vi "PPG_ABC.constructor.vi"(0 "name":string, 2 "data in":string, 5 "error in(no error)":errorcluster) -> (14 "i ref out":refnum<vi>, 16 "data out":string, 19 "error out":errorcluster)   [LabVIEW 2014, in "PPG_ABC.lvlib"]
doc: "This is the constructor of a class.\n\nLicense Agreement for this software:\n\nCopyright (C)\nGesellschaft für Schwerionenforschung, GSI\nPlanckstr. 1\n64291 Darmstadt\nGermany\n\nContact: D.Beck@gsi.de \n\nThis program is free software; you can redistribute it and/or modify it under the terms of the \nGNU General Public License as published by the Free Software Foundation; either version 2 of \nthe license, or (at your option) any later version.\n\nThis program is distributed in the hope that it will be useful, but WITHOUT ANY WARRANTY; \nwithout even the implied warranty of MERCHANTABILITY or FITNESS FOR A PARTICULAR PURPOSE. See the GNU General License for more details (http://www.gnu.org).\n\nGesellschaft für Schwerionenforschung, GSI\nPlanckstr. 1, 64291 Darmstadt, Germany\nFor all questions and ideas contact: M.Richter@gsi.de, H.Brand@gsi.de or D.Beck@gsi.de.\nLast update: 16-JUN-2004"
uses:
  PPG_ABC.lvlib
  CSCore/CSApplicationBaseClasses/DeviceBase/DeviceBase.myEventNames.ctl
  CSCore/CSSystem/CSSystemLib/CSSystemLib.lvlib
  CSCore/CSApplicationBaseClasses/DeviceBase/DeviceBase.lvlib
  NI_FPGA_PPG/NI_FPGA_PPG.lvlib
  CSlibraries-extern/DimLVEvent/LVDimInterface/LVDimInterface.lvlib
  CSCore/BaseProcess/BaseProcess.lvlib
  CSCore/CSObj/CSObj.lvlib
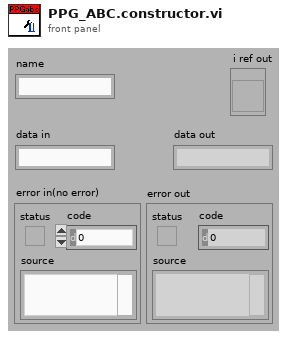
[diagram p1: front panel]
types:
  T1 = enum16{"SetAttribute", "GetAttribute", "CreateAttribute", "DestroyAttribute", "DestroyAllAtributes"}
  T2 = typedef "DeviceBase.lvlib/DeviceBase.myEventNames.ctl" = enum16{"lvmsg://Initialize", "lvmsg://Close", "lvmsg://Configure", "lvmsg://Reset", "lvmsg://IDQuery"}
  T3 = typedef "Semaphore RefNum" = refnum<k1>
  T4 = typedef "PPG_ABC.lvlib/PPG_ABC.i attribute.ctl" = cluster{"patternGroups":T5[], "defaultLetter":string, "defaultPatternGroup":i32, "PGRunning":T6, "PGRunningID":i32, "pgStarting":T3}
  T5 = typedef "PPG_ABC.lvlib/PPG_ABC.PG_dataType.ctl" = cluster{"PGDevice":string, "rawPatternData":cluster{"triggerCondition":i32, "timeTable":dbl[], "channelTable":string[]}[]}
  T6 = typedef "PPG_ABC.lvlib/PPG_ABC.PG_Running.ctl" = i32
  T7 = typedef "CSObj.lvlib/CSObj.i attribute.ctl" = cluster{"VI Refnum":refnum<vi>, "Front Panel Ref":refnum<vi>, "semaphore":T3, "date of birth":dbl, "ageID":i32, "systemID":i32, "classID":i32, "conditionID":i32, "DefaultPanelType":u16}
  T8 = typedef "BaseProcess.lvlib/BaseProcess.i attribute.ctl" = cluster{"EventStatus":string, "EventError":i32, "PresetEvtWatchD":i32, "PresetPdcWatchD":i32, "EventTimeout":i32, "PeriodicInterval":i32, "Interface":string[], "Address":string[], "Special":string[], "PeriodicError":i32, "PeriodicStatus":string, "SuperProc":string, "Descriptors":T9[], "CaseRef":refnum<vi>, "PdcRef":refnum<vi>, "Thread Ref":refnum<vi>, "eventErrorID":i32, "eventStatusID":i32, "periodicErrorID":i32, "periodicStatusID":i32, "pdcCtrID":i32}
  T9 = typedef "BaseProcess.lvlib/BaseProcess.descriptor definition.ctl" = cluster{"selector":string, "descriptor":T10}
  T10 = typedef "BaseProcess.lvlib/BaseProcess.descriptor string definition.ctl" = string
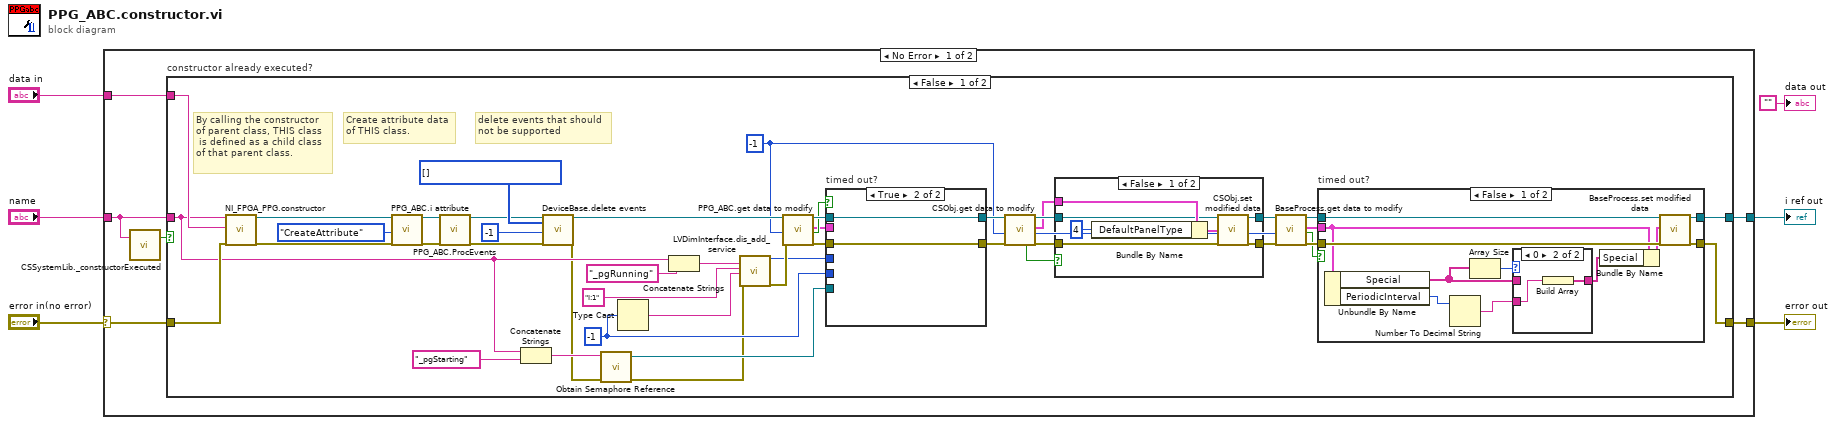
[diagram p0: block diagram]
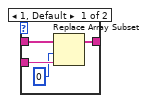
[diagram p3: hidden frame]
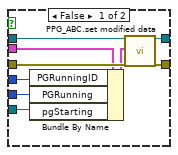
[diagram p5: hidden frame]
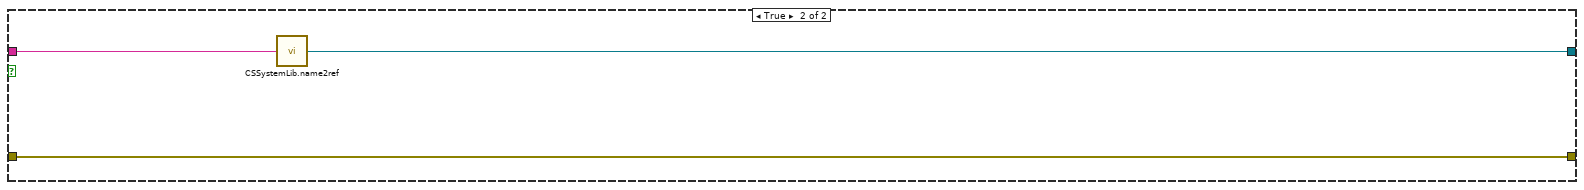
[diagram p6: hidden frame]
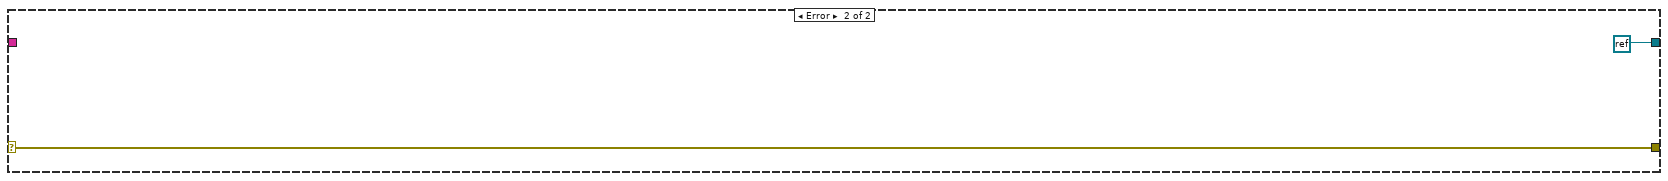
[diagram p7: hidden frame]
diagram:
  n1 = case shown="No Error" "error in(no error)" {
    selector: "error in(no error)" -> [w10 w99]
    tunnel: "name" -> [w9 _]
    tunnel: [w12 refnum<k0> refnum ("Not a Refnum Constant")] -> w5
    tunnel: [w11 w99] -> w4
    tunnel: "data in" -> [w7 _]
    frame No Error {
      n2 = call "CSSystemLib._constructorExecuted.vi"("name"=w9) -> ("constructor executed?"=w8:bool)  [unwired: 18 in]
      n3 = case "constructor already executed?" shown="False" w8 {
        tunnel: w9 -> [w26 w98]
        tunnel: [w29 w97] -> w12
        tunnel: [w28 w96] -> w11
        tunnel: w10 -> [w51 w96]
        tunnel: w7 -> [w46 _]
        frame False {
          w50 = T2[] [] items=["lvmsg://Initialize", "lvmsg://Close", "lvmsg://Configure", "lvmsg://Reset", "lvmsg://IDQuery"] ("events")
          w19 = -1 ("ms timeout (10000)")
          w34 = -1
          # "delete events that should\nnot be supported"
          # "Create attribute data\nof THIS class."
          # "By calling the constructor\nof parent class, THIS class\n is defined as a child class\nof that parent class."
          n4 = call "NI_FPGA_PPG.constructor.vi"("name"=w26, "data in"=w46, "error in (no error)"=w51) -> ("i ref out"=w56:refnum<vi>, "error out"=w55:errorcluster)  [unwired: 14 in, 1 out]
          n5 = call "PPG_ABC.i attribute.vi"("VI Refnum"=w56, "Action"=T1."CreateAttribute", "error in (no error)"=w55) -> ("VI Refnum out"=w53:refnum<vi>, "error out"=w52:errorcluster)  [unwired: 14 in, 1 out]
          n6 = call "PPG_ABC.ProcEvents.vi"("i ref in"=w53, "error in (no error)"=w52) -> ("i ref out"=w49:refnum<vi>, "error out"=w47:errorcluster)  [unwired: 16 in]
          n7 = Concatenate Strings(w26, "_pgStarting" ("string")) -> (w27:string)
          n8 = call "DeviceBase.delete events.vi"("i ref in"=w49, "events"=w50, "ms timeout (10000)"=-1, "error in (no error)"=w47) -> ("i ref out"=w41:refnum<vi>, "error out"=w23:errorcluster)  [unwired: 13 in, 1 out]
          n9 = call <vilib>:"Obtain Semaphore Reference.vi"("error in (no error)"=w23, "name (unnamed)"=w27) -> ("error out"=w22:errorcluster, "semaphore"=w24:T3)  [unwired: 3 in, 1 out]
          n10 = Type Cast(x=w34) -> (*(type *) &x=w42:string)  [unwired: 1 in]
          n11 = Concatenate Strings(w26, "_pgRunning" ("string")) -> (w44:string)
          n12 = call "LVDimInterface.dis_add_service.vi"("serviceName"=w44, "typeDescriptor"="I:1", "data"=w42, "error in (no error)"=w22) -> ("my_serviceID"=w35:i32, "error out"=w40:errorcluster)  [unwired: 14 in]
          n13 = call "PPG_ABC.get data to modify.vi"("i ref in"=w41, "ms timeout (10000)"=w19, "error in (no error)"=w40) -> ("i ref out"=w39:refnum<vi>, "i attribute"=w36:T4, "timed out"=w38:bool, "error out"=w37:errorcluster)  [unwired: 13 in]
          n14 = case "timed out?" shown="True" w38 {
            tunnel: w39 -> [w93 w95]
            tunnel: w37 -> [w92 w94]
            tunnel: w36 -> [w91 _]
            tunnel: w35 -> [w90 _]
            tunnel: w34 -> [w89 _]
            tunnel: [w88 w95] -> w21
            tunnel: [w87 w94] -> w20
            tunnel: w24 -> [w85 _]
            frame False {
              n15 = Bundle By Name(cluster=w91, "PGRunningID"=w90, "PGRunning"=w89, "pgStarting"=w85) -> (w86:T4)
              n16 = call "PPG_ABC.set modified data.vi"("i ref in"=w93, "i attribute"=w86, "error in (no error)"=w92) -> ("i ref out"=w88:refnum<vi>, "error out"=w87:errorcluster)  [unwired: 15 in]
            }
            frame True {
            }
          }
          n17 = call "CSObj.get data to modify.vi"("i ref in"=w21, "error in (no error)"=w20) -> ("i ref out"=w16:refnum<vi>, "i attribute"=w13:T7, "timed out"=w18:bool, "error out"=w14:errorcluster)  [unwired: 14 in]
          n18 = case shown="False" w18 {
            tunnel: [w61 w65] -> w17
            tunnel: w16 -> [w62 w65]
            tunnel: [w59 w64] -> w15
            tunnel: w14 -> [w60 w64]
            tunnel: w13 -> [w63 _]
            frame False {
              n19 = Bundle By Name(cluster=w63, "DefaultPanelType"=u16 4) -> (w58:T7)
              n20 = call "CSObj.set modified data.vi"("i ref in"=w62, "i attribute"=w58, "error in (no error)"=w60) -> ("i ref out"=w61:refnum<vi>, "error out"=w59:errorcluster)  [unwired: 15 in]
            }
            frame True {
            }
          }
          n21 = call "BaseProcess.get data to modify.vi"("i ref in"=w17, "ms timeout (10000)"=w19, "error in (no error)"=w15) -> ("i ref out"=w33:refnum<vi>, "i attribute"=w32:T8, "timed out"=w30:bool, "error out"=w31:errorcluster)  [unwired: 13 in]
          n22 = case "timed out?" shown="False" w30 {
            tunnel: w33 -> [w76 w84]
            tunnel: w31 -> [w75 w83]
            tunnel: w32 -> [w71 _]
            tunnel: [w74 w84] -> w29
            tunnel: [w73 w83] -> w28
            frame False {
              n23 = Unbundle By Name(w71) -> ("Special"=w66:string[], "PeriodicInterval"=w70:i32)
              n24 = Number To Decimal String(number=w70) -> (decimal integer string=w69:string)  [unwired: 1 in]
              n25 = Array Size(array=w66) -> (size(s)=w67:i32)
              n26 = case shown="0" w67 {
                tunnel: w69 -> [w78 w82]
                tunnel: [w79 w81] -> w68
                tunnel: w66 -> [w80 _]
                frame 1, Default {
                  n27 = Replace Array Subset(array=w80, new element=w78, index=0) -> (w79:string[])
                }
                frame 0 {
                  n28 = Build Array(w82) -> (w81:string[])
                }
              }
              n29 = Bundle By Name(cluster=w71, "Special"=w68) -> (w72:T8)
              n30 = call "BaseProcess.set modified data.vi"("i ref in"=w76, "i attribute"=w72, "error in (no error)"=w75) -> ("i ref out"=w74:refnum<vi>, "error out"=w73:errorcluster)  [unwired: 15 in]
            }
            frame True {
            }
          }
        }
        frame True {
          n31 = call "CSSystemLib.name2ref.vi"("name"=w98) -> ("obj refnum"=w97:refnum<vi>)
        }
      }
    }
    frame Error {
    }
  }
  "i ref out" <- w5
  "error out" <- w4
  "data out" <- "" ("Empty String Constant")
